vi "Delay (SubVI).vi"(11 "delay":fxp<+/-,16,4>) -> (3 "g 2":fxp<+/-,16,4>)   [LabVIEW 2016]
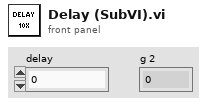
[diagram p1: front panel]
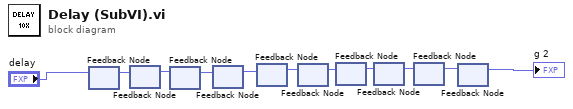
[diagram p0: block diagram]
diagram:
  n1 = feedback #1() -> (w1:fxp<+/-,16,4>)  [unwired: 1 in]
  n2 = feedback-in #1("delay") -> ()
  n3 = feedback #2() -> (w2:fxp<+/-,16,4>)  [unwired: 1 in]
  n4 = feedback-in #2(w1) -> ()
  n5 = feedback #3() -> (w3:fxp<+/-,16,4>)  [unwired: 1 in]
  n6 = feedback-in #3(w2) -> ()
  n7 = feedback #4() -> (w4:fxp<+/-,16,4>)  [unwired: 1 in]
  n8 = feedback-in #4(w3) -> ()
  n9 = feedback #5() -> (w5:fxp<+/-,16,4>)  [unwired: 1 in]
  n10 = feedback-in #5(w4) -> ()
  n11 = feedback #6() -> (w6:fxp<+/-,16,4>)  [unwired: 1 in]
  n12 = feedback-in #6(w5) -> ()
  n13 = feedback #7() -> (w7:fxp<+/-,16,4>)  [unwired: 1 in]
  n14 = feedback-in #7(w6) -> ()
  n15 = feedback #8() -> (w8:fxp<+/-,16,4>)  [unwired: 1 in]
  n16 = feedback-in #8(w7) -> ()
  n17 = feedback #9() -> (w9:fxp<+/-,16,4>)  [unwired: 1 in]
  n18 = feedback-in #9(w8) -> ()
  n19 = feedback #10() -> (→"g 2":fxp<+/-,16,4>)  [unwired: 1 in]
  n20 = feedback-in #10(w9) -> ()
